vi "Initialize_Control_Brass.vi"(0 "ERD Loop":refnum<queue>, 2 "GEA2":refnum<queue>, 5 "Receive Loop":refnum<user-event>, 7 "UI Loop Error":refnum<user-event>, 9 "Cont Send":refnum<queue>, 11 "Error In":errorcluster, 13 "DAQ":refnum<queue>) -> (15 "Error Out":errorcluster)   [LabVIEW 2016]
uses:
  type defs2/ERD_Data_Loop_Control_Brass.ctl
  type defs2/ERD_Loop_States_Brass.ctl
  Common/GExplorer Support/typedefs/GExplorer_Data_Cluster.ctl
  type defs2/DAQ_States_Brass.ctl
  type defs2/Cont_Send_States_Brass.ctl
  type defs2/Error_Command_Brass.ctl
  type defs2/ERD_Loop_Control_Command_Brass.ctl
  type defs2/DAQ_Control_Command_Brass.ctl
  type defs2/GEA2_Control_Command_Brass.ctl
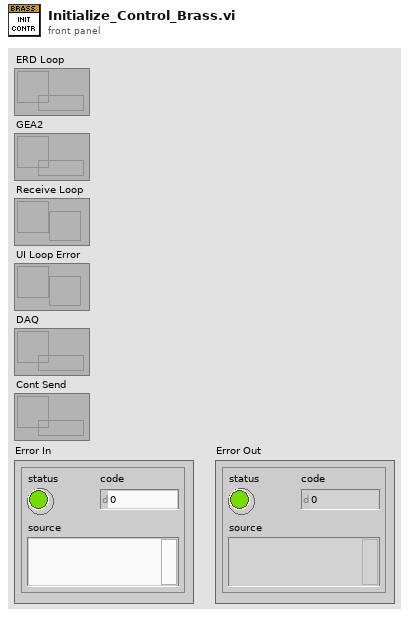
[diagram p1: front panel]
types:
  T1 = typedef "GEA2_Control_Command_Brass.ctl" = enum16{"Initialize", "Shutdown"}
  T2 = typedef "DAQ_Control_Command_Brass.ctl" = enum16{"Initialize", "Shutdown", "Exit"}
  T3 = typedef "ERD_Loop_Control_Command_Brass.ctl" = enum16{"Initialize", "Shutdown"}
  T4 = typedef "Error_Command_Brass.ctl" = enum16{"Initialize", "Handle Errors", "Report Errors"}
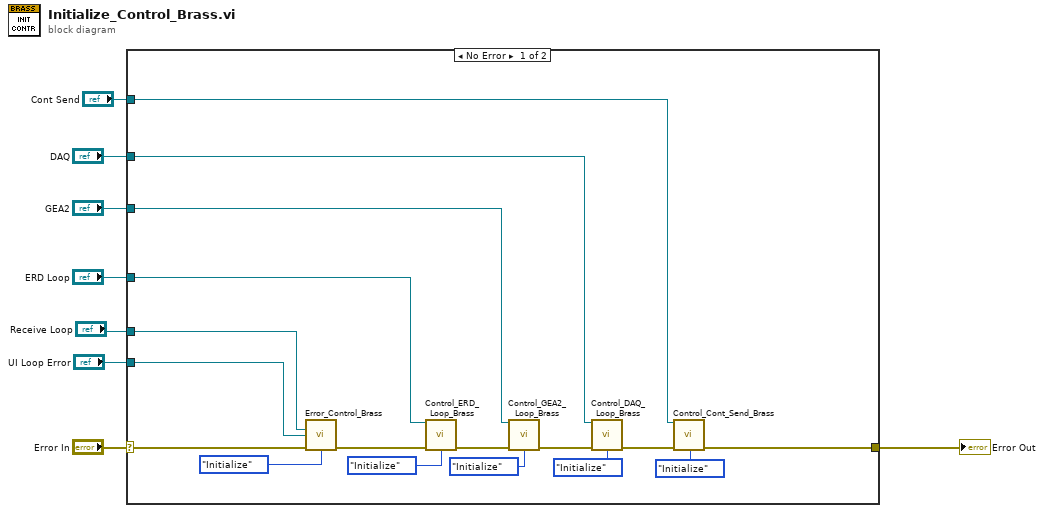
[diagram p0: block diagram]
diagram:
  n1 = case shown="No Error" "Error In" {
    selector: "Error In" -> [w19 w26]
    tunnel: [w11 w26] -> w7
    tunnel: "Receive Loop" -> [w13 _]
    tunnel: "ERD Loop" -> [w18 _]
    tunnel: "GEA2" -> [w17 _]
    tunnel: "DAQ" -> [w15 _]
    tunnel: "UI Loop Error" -> [w14 _]
    tunnel: "Cont Send" -> [w9 _]
    frame No Error {
      n2 = call "Error_Control_Brass.vi"("Command (Handle Errors)"=Error_Command_Brass."Initialize", "Receive Loop"=w13, "UI Loop Error"=w14, "Error In"=w19) -> ("Error Out"=w20:errorcluster)  [unwired: 11 in]
      n3 = call "Control_ERD_Loop_Brass.vi"("ERD Loop"=w18, "Command (ERD Loop Control)"=ERD_Loop_Control_Command_Brass."Initialize", "Error In"=w20) -> ("Error Out"=w23:errorcluster)  [unwired: 12 in]
      n4 = call "Control_GEA2_Loop_Brass.vi"("GEA2"=w17, "Command (ERD Loop Control)"=GEA2_Control_Command_Brass."Initialize", "Error In"=w23) -> ("Error Out"=w21:errorcluster)  [unwired: 12 in]
      n5 = call "Control_DAQ_Loop_Brass.vi"("DAQ"=w15, "Command (DAQ Control)"=DAQ_Control_Command_Brass."Initialize", "Error In"=w21) -> ("Error Out"=w12:errorcluster)  [unwired: 12 in]
      n6 = call "Control_Cont_Send_Brass.vi"("Cont Send"=w9, "Command (ERD Loop Control)"=GEA2_Control_Command_Brass."Initialize", "Error In"=w12) -> ("Error Out"=w11:errorcluster)  [unwired: 12 in]
    }
    frame Error {
    }
  }
  "Error Out" <- w7
